vi "2283_gyroPID.vi"(0 "Gyro Input":dbl, 1 "Gyro Boolean":bool, 2 "Angulo":dbl format="%#_13g", 3 "Angulo Deseado":dbl format="%#_13g") -> (5 "Gyro Output":dbl(slide) scale=-5000.0..5000.0)   [LabVIEW 2014]
uses:
  <vilib>/addons/control/pid/pid.llb/PID (DBL).vi
  <vilib>/addons/control/pid/NI_PID_pid.lvlib
panel:
  in  "PID gains":T1={"proportional gain (Kc)"=180.0, "integral time (Ti, min)"=2e-05, "derivative time (Td, min)"=3.0}
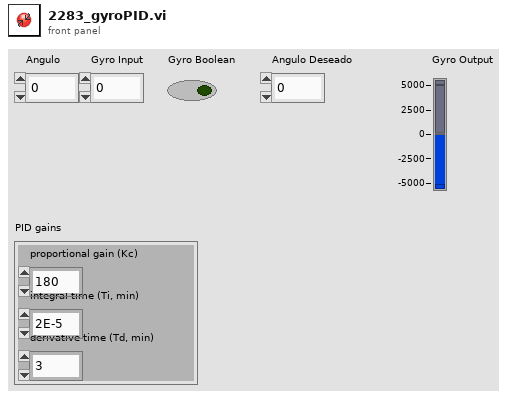
[diagram p1: front panel]
types:
  T1 = cluster{"proportional gain (Kc)":dbl, "integral time (Ti, min)":dbl, "derivative time (Td, min)":dbl}
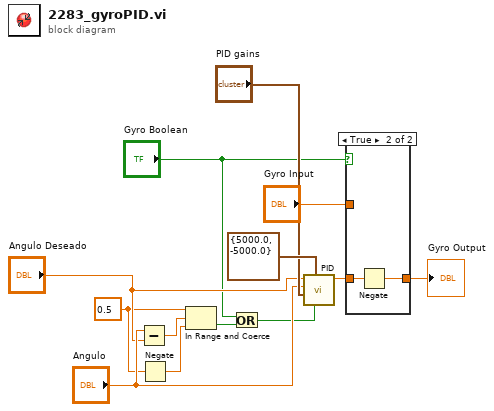
[diagram p0: block diagram]
diagram:
  w4 = 0.5
  n1 = Subtract(x="Angulo", y="Angulo Deseado") -> (x-y=w8:dbl)
  n2 = Negate(x=w4) -> (-x=w5:dbl)
  n3 = In Range and Coerce(upper limit=w4, x=w8, lower limit=w5) -> (In Range?=w2:bool)  [unwired: 1 out]
  n4 = Or(x="Gyro Boolean", y=w2) -> (x .or. y?=w3:bool)
  n5 = call-poly <vilib>:"PID.vi"("reinitialize? (F)"=w3, "output range"=cluster{"output high":dbl, "output low":dbl} {"output high"=5000.0, "output low"=-5000.0}, "PID gains"="PID gains", "process variable"="Angulo", "setpoint"="Angulo Deseado") -> ("output"=w10:dbl)  [unwired: 5 in, 1 out]
  n6 = case shown="True" "Gyro Boolean" {
    tunnel: [w14 w15] -> w12
    tunnel: w10 -> [_ w16]
    tunnel: "Gyro Input" -> [w14 _]
    frame False {
    }
    frame True {
      n7 = Negate(x=w16) -> (-x=w15:dbl)
    }
  }
  "Gyro Output" <- w12
